vi "Labspec Template.vi"(6 "Value":variant, 7 "Template Name":string, 8 "error in":errorcluster, 9 "Parameter":T1, 10 "Mode":T2, 11 "Automation Refnum In":refnum<k7>) -> (0 "error out":errorcluster, 1 "pValue":variant, 3 "Automation Refnum Out":refnum<k7>)   [LabVIEW 2014]
uses:
  NGSLabspec/NGSLabSpec.llb/Template Mode.ctl
  NGSLabspec/NGSLabSpec.llb/Template Parameter.ctl
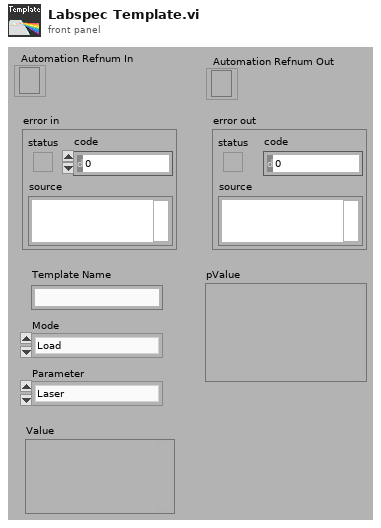
[diagram p1: front panel]
types:
  T1 = typedef "Template Parameter.ctl" = enum16{"Laser", "Filter", "Accumulation", "Spike", "Auto Exposure", "Auto Focus", "Grating", "Raman Polarizer", "Laser Polarizer", "Central Position", "Position From", "Position To", "Exposition", "Hole", "Slit", "AutoExposure Min", "AutoExposure Max", "Extended Range", "Objective"}
  T2 = typedef "Template Mode.ctl" = enum16{"Load", "Save", "Add To List", "Set Value", "Get Value", "Apply ", "Get Status", "Save Current Config", "Test", "Apply No Spectro"}
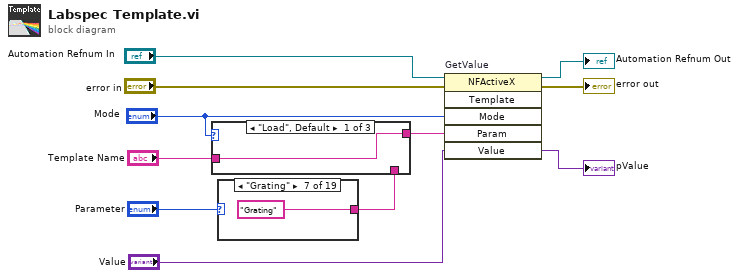
[diagram p0: block diagram]
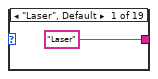
[diagram p4: hidden frame]
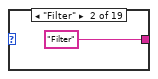
[diagram p5: hidden frame]
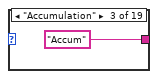
[diagram p6: hidden frame]
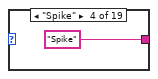
[diagram p7: hidden frame]
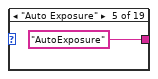
[diagram p8: hidden frame]
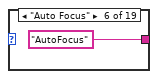
[diagram p9: hidden frame]
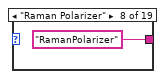
[diagram p10: hidden frame]
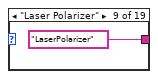
[diagram p11: hidden frame]
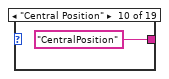
[diagram p12: hidden frame]
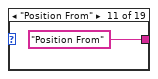
[diagram p13: hidden frame]
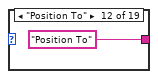
[diagram p14: hidden frame]
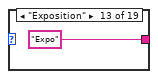
[diagram p15: hidden frame]
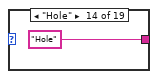
[diagram p16: hidden frame]
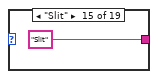
[diagram p17: hidden frame]
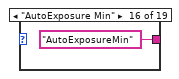
[diagram p18: hidden frame]
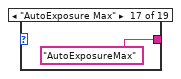
[diagram p19: hidden frame]
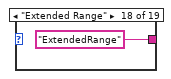
[diagram p20: hidden frame]
diagram:
  n1 = case shown="\"Grating\"" "Parameter" {
    tunnel: ["Laser" "Filter" "Accum" "Spike" "AutoExposure" "AutoFocus" "Grating" "RamanPolarizer" "LaserPolarizer" "CentralPosition" "Position From" "Position To" "Expo" "Hole" "Slit" "AutoExposureMin" "AutoExposureMax" "ExtendedRange" "Objective"] -> w3
    frame "Laser", Default {
    }
    frame "Filter" {
    }
    frame "Accumulation" {
    }
    frame "Spike" {
    }
    frame "Auto Exposure" {
    }
    frame "Auto Focus" {
    }
    frame "Grating" {
    }
    frame "Raman Polarizer" {
    }
    frame "Laser Polarizer" {
    }
    frame "Central Position" {
    }
    frame "Position From" {
    }
    frame "Position To" {
    }
    frame "Exposition" {
    }
    frame "Hole" {
    }
    frame "Slit" {
    }
    frame "AutoExposure Min" {
    }
    frame "AutoExposure Max" {
    }
    frame "Extended Range" {
    }
    frame "Objective" {
    }
  }
  n2 = case shown="\"Load\", Default" "Mode" {
    tunnel: [w31 w32 w33] -> w4
    tunnel: w3 -> [_ w32 w33]
    tunnel: "Template Name" -> [w31 _ _]
    frame "Load", Default {
    }
    frame "Set Value" {
    }
    frame "Get Value" {
    }
  }
  n3 = invoke on="GetValue" class="NFActiveX" method="Template"(reference="Automation Refnum In", error in="error in", "Mode"="Mode", "Param"=w4, "Value"="Value") -> (reference out=→"Automation Refnum Out":refnum<k7>, error out=→"error out":errorcluster, "Value"=→"pValue":variant)  [unwired: 1 in, 3 out]
